vi "IncorrectResponse.vi"(8 "error in (no error)":errorcluster, 11 "TrialBasedExperiment in":refnum<class "ClassDiscrimination.lvclass">) -> (0 "error out":errorcluster, 3 "TrialBasedExperiment out":refnum<class "ClassDiscrimination.lvclass">)   [LabVIEW 2014, in "ClassDiscrimination.lvclass"]
uses:
  ClassDiscrimination.lvclass
  ClassDiscrimination.lvclass/ClassDiscrimination.ctl
  Trial Based Experiment Statechart/MatlabExperiment/MatlabExperiment.lvclass
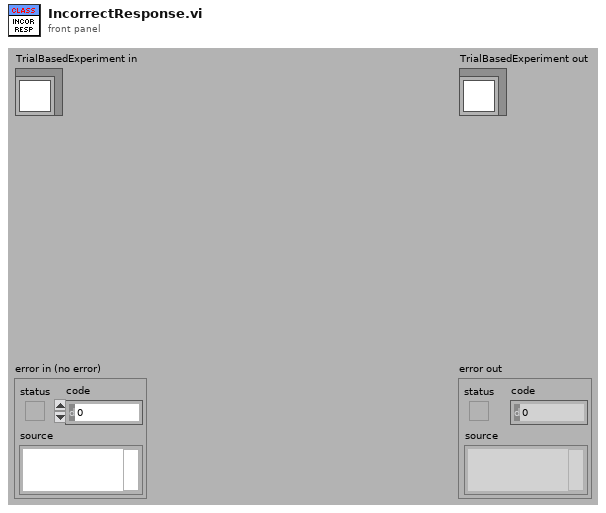
[diagram p1: front panel]
types:
  T1 = cluster{"Intertrial":dbl, "AcquireFixation":dbl, "HoldFixation":dbl, "DelayPeriod":dbl, "ResponsePeriod":dbl}
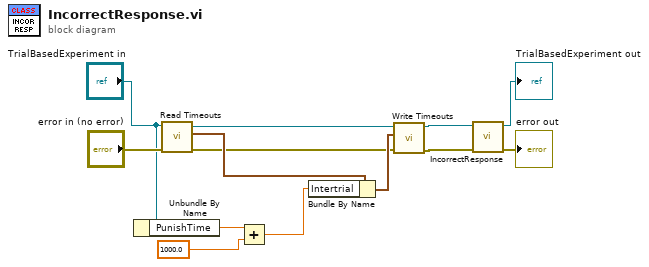
[diagram p0: block diagram]
diagram:
  n1 = Unbundle By Name("TrialBasedExperiment in") -> ("PunishTime"=w1:dbl)
  n2 = call-dynamic "Read Timeouts.vi"("error in (no error)"="error in (no error)", "TrialBasedExperiment in"="TrialBasedExperiment in") -> ("error out"=w8:errorcluster, "Timeouts"=w11:T1, "TrialBasedExperiment out"=w9:refnum<class "ClassDiscrimination.lvclass">)  [unwired: 7 in]
  n3 = Add(x=w1, y=1000.0 ("Intertrial")) -> (x+y=w3:dbl)
  n4 = Bundle By Name(cluster=w11, "Intertrial"=w3) -> (w10:T1)
  n5 = call-dynamic "Write Timeouts.vi"("error in (no error)"=w8, "Timeouts"=w10, "TrialBasedExperiment in"=w9) -> ("error out"=w6:errorcluster, "TrialBasedExperiment out"=w5:refnum<class "ClassDiscrimination.lvclass">)  [unwired: 7 in]
  n6 = call-parent "IncorrectResponse.vi"("error in (no error)"=w6, "TrialBasedExperiment in"=w5) -> ("error out"=→"error out":errorcluster, "TrialBasedExperiment out"=→"TrialBasedExperiment out":refnum<class "ClassDiscrimination.lvclass">)  [unwired: 8 in]
